vi "ShooterState.vi"() -> ()   [LabVIEW 2019]
panel:
  out "ShooterReady":bool
  out "Aimed":bool
  out "TargetAcquired":bool
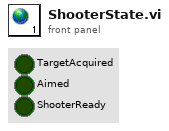
[diagram p1: front panel]
diagram:
